vi "Kiwi_Get_Set_Refnum.vi"(8 "error in (no error)":errorcluster, 9 "menu":T11=enum."get", 10 "refnum name":string, 11 "Kiwi DevRef In":T1={"Motor A"={"DeviceStatus"={"status"=FALSE, "code"=0, "source"=""}, "Type"=enum."PWM", "PWM"={"PWM Channel"=enum."Invalid", "DeadBand"={"Name"="", "maxPositivePwm"=0, "minPositivePwm"=0, "centerPwm"=0, "maxNegativePwm"=0, "minNegativePwm"=0, "angularRange"=0}}, "CAN"={"Device Number"=0, "Control Mode"=enum."Percent VBus", "Semaphore"=refnum, "Max Vout"=12.0, "TalonSRX Control Mode"=enum."Percent VBus"}, "Invert"=FALSE}, "Motor B"={"DeviceStatus"={"status"=FALSE, "code"=0, "source"=""}, "Type"=enum."PWM", "PWM"={"PWM Channel"=enum."Invalid", "DeadBand"={"Name"="", "maxPositivePwm"=0, "minPositivePwm"=0, "centerPwm"=0, "maxNegativePwm"=0, "minNegativePwm"=0, "angularRange"=0}}, "CAN"={"Device Number"=0, "Control Mode"=enum."Percent VBus", "Semaphore"=refnum, "Max Vout"=12.0, "TalonSRX Control Mode"=enum."Percent VBus"}, "Invert"=FALSE}, "Motor C"={"DeviceStatus"={"status"=FALSE, "code"=0, "source"=""}, "Type"=enum."PWM", "PWM"={"PWM Channel"=enum."Invalid", "DeadBand"={"Name"="", "maxPositivePwm"=0, "minPositivePwm"=0, "centerPwm"=0, "maxNegativePwm"=0, "minNegativePwm"=0, "angularRange"=0}}, "CAN"={"Device Number"=0, "Control Mode"=enum."Percent VBus", "Semaphore"=refnum, "Max Vout"=12.0, "TalonSRX Control Mode"=enum."Percent VBus"}, "Invert"=FALSE}, "Config Consts"={"Arx"=0.0, "Ay"=0.0, "Brx"=0.0, "By"=0.0, "Cr"=0.0, "Cy"=0.0, "Cx"=0.0, "MaxMotorVal"=0.0}, "status"={"status"=FALSE, "code"=0, "source"=""}, "Angles"={"Angle A"=60.0, "Angle B"=60.0, "Angle C"=60.0, "Radians?"=FALSE}, "MotorVals"={"MotorA"=0.0, "MotorB"=0.0, "MotorC"=0.0}}) -> (0 "error out":errorcluster, 2 "Kiwi DevRef Out":T1={"Motor A"={"DeviceStatus"={"status"=FALSE, "code"=0, "source"=""}, "Type"=enum."PWM", "PWM"={"PWM Channel"=enum."Invalid", "DeadBand"={"Name"="", "maxPositivePwm"=0, "minPositivePwm"=0, "centerPwm"=0, "maxNegativePwm"=0, "minNegativePwm"=0, "angularRange"=0}}, "CAN"={"Device Number"=0, "Control Mode"=enum."Percent VBus", "Semaphore"=refnum, "Max Vout"=12.0, "TalonSRX Control Mode"=enum."Percent VBus"}, "Invert"=FALSE}, "Motor B"={"DeviceStatus"={"status"=FALSE, "code"=0, "source"=""}, "Type"=enum."PWM", "PWM"={"PWM Channel"=enum."Invalid", "DeadBand"={"Name"="", "maxPositivePwm"=0, "minPositivePwm"=0, "centerPwm"=0, "maxNegativePwm"=0, "minNegativePwm"=0, "angularRange"=0}}, "CAN"={"Device Number"=0, "Control Mode"=enum."Percent VBus", "Semaphore"=refnum, "Max Vout"=12.0, "TalonSRX Control Mode"=enum."Percent VBus"}, "Invert"=FALSE}, "Motor C"={"DeviceStatus"={"status"=FALSE, "code"=0, "source"=""}, "Type"=enum."PWM", "PWM"={"PWM Channel"=enum."Invalid", "DeadBand"={"Name"="", "maxPositivePwm"=0, "minPositivePwm"=0, "centerPwm"=0, "maxNegativePwm"=0, "minNegativePwm"=0, "angularRange"=0}}, "CAN"={"Device Number"=0, "Control Mode"=enum."Percent VBus", "Semaphore"=refnum, "Max Vout"=12.0, "TalonSRX Control Mode"=enum."Percent VBus"}, "Invert"=FALSE}, "Config Consts"={"Arx"=0.0, "Ay"=0.0, "Brx"=0.0, "By"=0.0, "Cr"=0.0, "Cy"=0.0, "Cx"=0.0, "MaxMotorVal"=0.0}, "status"={"status"=FALSE, "code"=0, "source"=""}, "Angles"={"Angle A"=60.0, "Angle B"=60.0, "Angle C"=60.0, "Radians?"=FALSE}, "MotorVals"={"MotorA"=0.0, "MotorB"=0.0, "MotorC"=0.0}}, 3 "refnum names":string[](array[string]))   [LabVIEW 2015]
uses:
  <vilib>/Rock Robotics/WPI/Utilities/Refnum Registry Operation.ctl
  <userlib>/836-Library/Drive/kiwi/support/Kiwi_Dev_Ref.ctl
  <vilib>/Rock Robotics/WPI/MotorControl/WPI_MotorControlDeviceRef.ctl
  <vilib>/Rock Robotics/WPI/MotorControl/WPI_MotorControlType.ctl
  <vilib>/Rock Robotics/SystemInterfaces/DIO/FPGA_DIOPWMChannel.ctl
  <vilib>/Rock Robotics/WPI/PWM/WPI_PWMDeadband.ctl
  <vilib>/Rock Robotics/WPI/CAN/Jaguar/SubVIs/WPI_CANJaguar_ControlMode.ctl
  <vilib>/Rock Robotics/WPI/CAN/TalonSRX/WPI_CANTalonSRX_APIControlMode.ctl
  <userlib>/836-Library/Drive/kiwi/support/Kiwi_Cal_Constants.ctl
  <userlib>/836-Library/Drive/kiwi/support/Kiwi_Angles.ctl
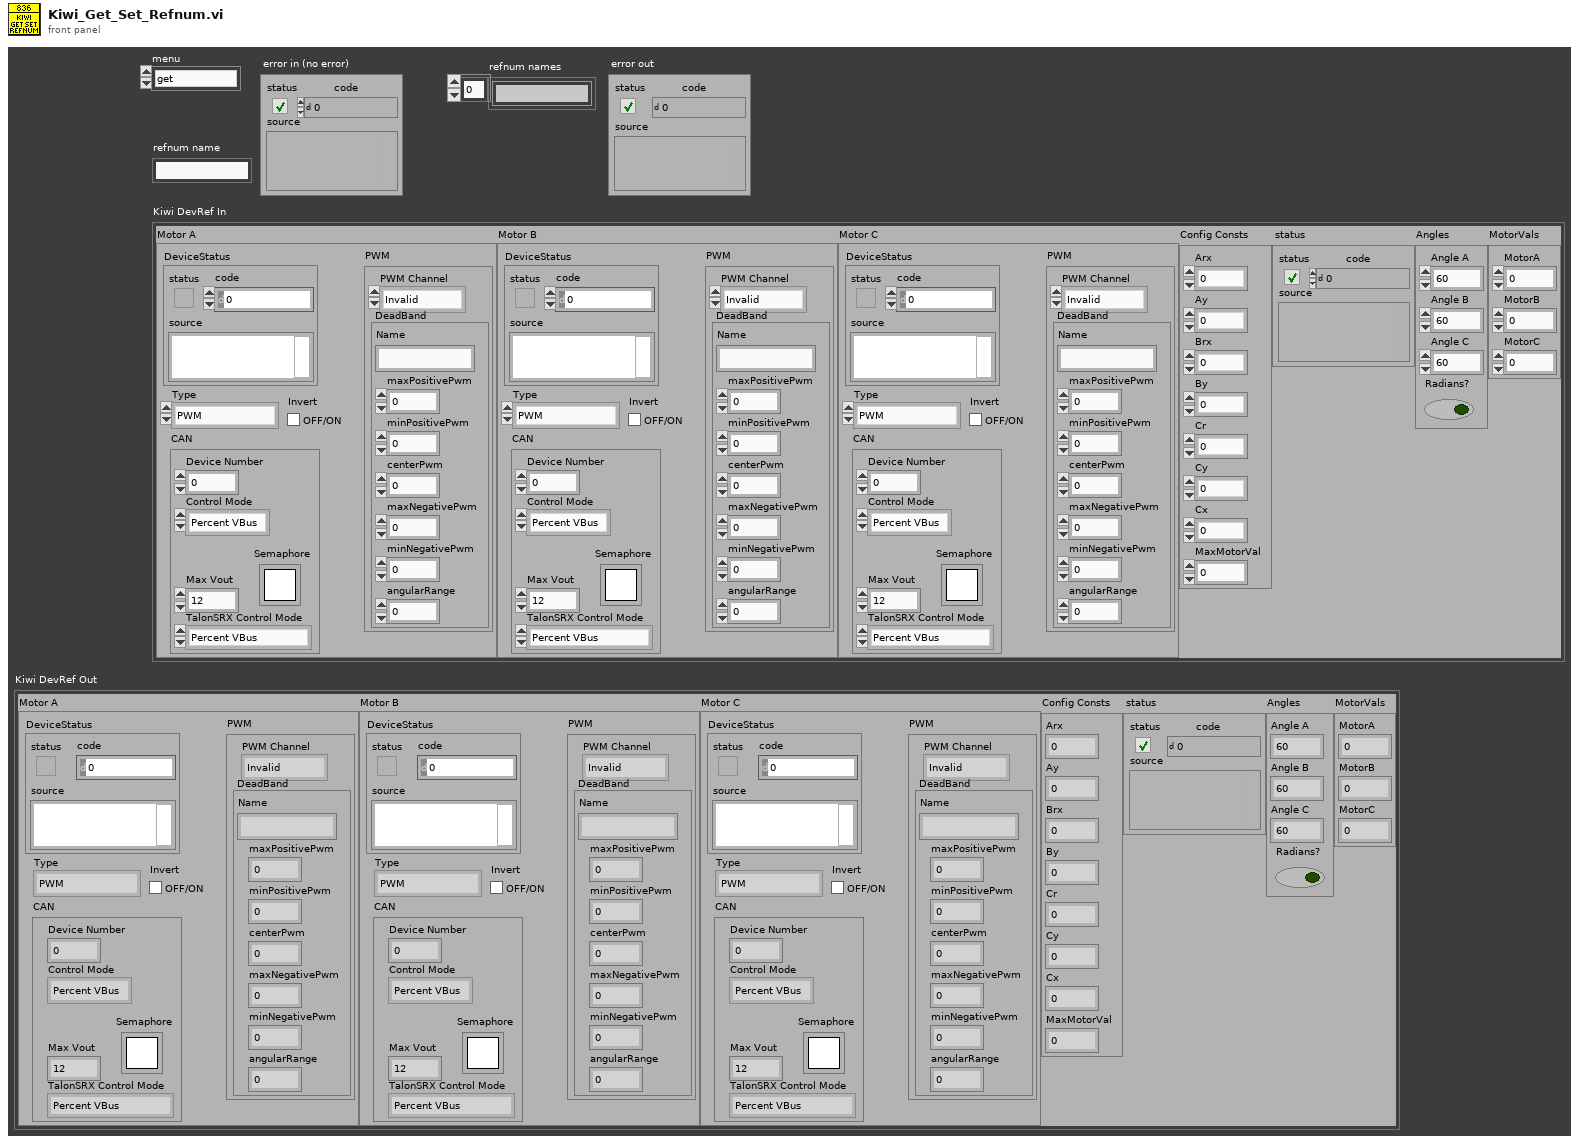
[diagram p1: front panel]
types:
  T1 = typedef "Kiwi_Dev_Ref.ctl" = cluster{"Motor A":T2, "Motor B":T2, "Motor C":T2, "Config Consts":T9, "status":errorcluster, "Angles":T10, "MotorVals":cluster{"MotorA":dbl, "MotorB":dbl, "MotorC":dbl}}
  T2 = typedef "WPI_MotorControlDeviceRef.ctl" = cluster{"DeviceStatus":errorcluster, "Type":T3, "PWM":cluster{"PWM Channel":T4, "DeadBand":T5}, "CAN":cluster{"Device Number":u8, "Control Mode":T6, "Semaphore":T7, "Max Vout":dbl, "TalonSRX Control Mode":T8}, "Invert":bool}
  T3 = typedef "WPI_MotorControlType.ctl" = enum16{"PWM", "CAN", "CANTalonSRX"}
  T4 = typedef "FPGA_DIOPWMChannel.ctl" = enum8{"PWM 0", "PWM 1", "PWM 2", "PWM 3", "PWM 4", "PWM 5", "PWM 6", "PWM 7", "PWM 8", "PWM 9", "PWM MXP 0", "PWM MXP 1", "PWM MXP 2", "PWM MXP 3", "PWM MXP 4", "PWM MXP 5", "PWM MXP 6", "PWM MXP 7", "PWM MXP 8", "PWM MXP 9", "Invalid"}
  T5 = typedef "WPI_PWMDeadband.ctl" = cluster{"Name":string, "maxPositivePwm":i32, "minPositivePwm":i32, "centerPwm":i32, "maxNegativePwm":i32, "minNegativePwm":i32, "angularRange":u16}
  T6 = typedef "WPI_CANJaguar_ControlMode.ctl" = enum8{"Percent VBus", "Current", "Speed", "Position", "Voltage"}
  T7 = typedef "Semaphore RefNum" = refnum<k1>
  T8 = typedef "WPI_CANTalonSRX_APIControlMode.ctl" = enum8{"Percent VBus", "Speed", "Position", "Slave", "Unchanged / Invalid", "Voltage Compensation", "Current", "Motion Profile"}
  T9 = typedef "Kiwi_Cal_Constants.ctl" = cluster{"Arx":dbl, "Ay":dbl, "Brx":dbl, "By":dbl, "Cr":dbl, "Cy":dbl, "Cx":dbl, "MaxMotorVal":dbl}
  T10 = typedef "Kiwi_Angles.ctl" = cluster{"Angle A":dbl, "Angle B":dbl, "Angle C":dbl, "Radians?":bool}
  T11 = typedef "Refnum Registry Operation.ctl" = enum16{"set", "get", "delete", "get all names", "read name"}
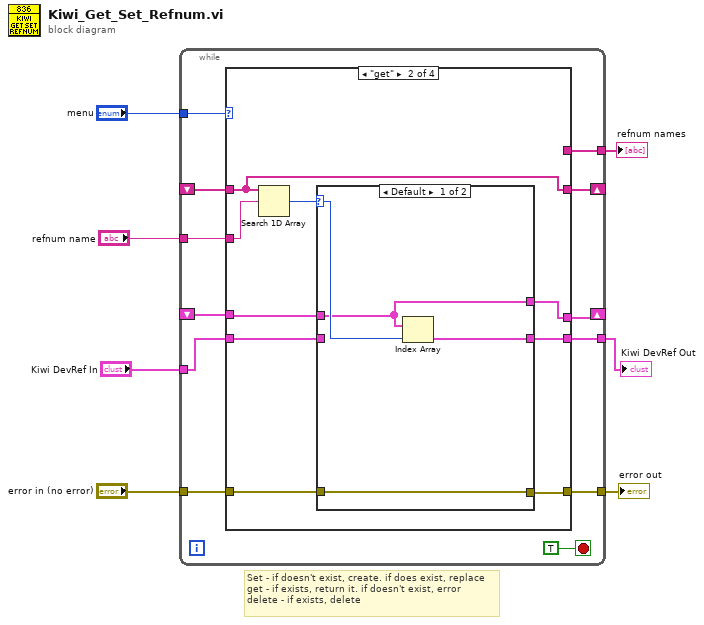
[diagram p0: block diagram]
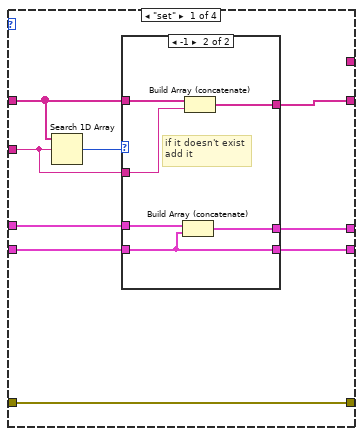
[diagram p2: hidden frame]
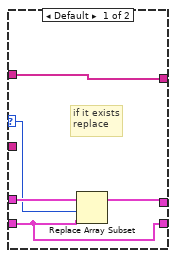
[diagram p3: hidden frame]
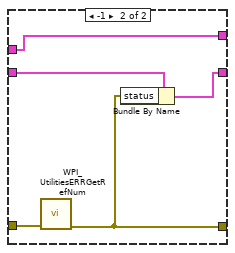
[diagram p4: hidden frame]
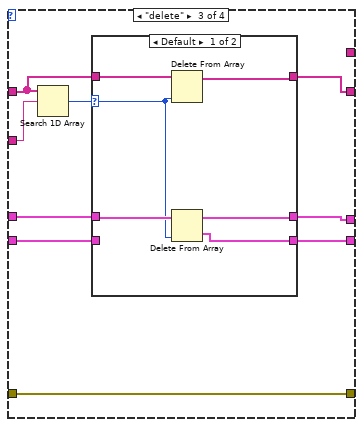
[diagram p5: hidden frame]
diagram:
  # "Set - if doesn't exist, create. if does exist, replace\nget - if exists, return it. if doesn't exist, error\ndelete - if exists, delete"
  n1 = while {
    tunnel: "menu" -> [w18]
    tunnel: "Kiwi DevRef In" -> [w11]
    tunnel: "refnum name" -> [w15]
    tunnel: "error in (no error)" -> [w16]
    shift-right: [w13] -> _
    shift-left: _ -> [w14]
    shift-right: [w9] -> _
    shift-left: _ -> [w12]
    tunnel: [w17] -> w3
    tunnel: [w10] -> w2
    tunnel: [w8] -> w1
    stop <- TRUE stop-if-true
    n2 = case shown="\"get\"" w18 {
      tunnel: [w21 w40 w66 w79] -> w17
      tunnel: w16 -> [w21 w42 w66 w79]
      tunnel: w15 -> [w28 w48 w65 _]
      tunnel: w14 -> [w20 w46 w62 w78]
      tunnel: [w27 w46 w63 w78] -> w13
      tunnel: w12 -> [w25 w45 w60 w77]
      tunnel: w11 -> [w24 w41 w58 w76]
      tunnel: [w23 w44 w59 w76] -> w10
      tunnel: [w22 w43 w61 w77] -> w9
      tunnel: [_ _ _ w78] -> w8
      frame "set" {
        n3 = Search 1D Array(1D array=w20, element=w28) -> (index of element=w26:i32)  [unwired: 1 in]
        n4 = case shown="-1" w26 {
          selector: w26 -> [w31 _]
          tunnel: w20 -> [w33 w39]
          tunnel: w28 -> [_ w38]
          tunnel: [w33 w37] -> w27
          tunnel: w25 -> [w32 w36]
          tunnel: w24 -> [w29 w35]
          tunnel: [w29 w35] -> w23
          tunnel: [w30 w34] -> w22
          frame Default {
            # "if it exists\nreplace"
            n5 = Replace Array Subset(array=w32, new element=w29, index=w31) -> (w30:T1[])
          }
          frame -1 {
            # "if it doesn't exist\nadd it"
            n6 = Build Array (concatenate)(w36, w35) -> (w34:T1[])
            n7 = Build Array (concatenate)(w39, w38) -> (w37:string[])
          }
        }
      }
      frame "get" {
        n8 = Search 1D Array(1D array=w46, element=w48) -> (index of element=w47:i32)  [unwired: 1 in]
        n9 = case shown="Default" w47 {
          selector: w47 -> [w52 _]
          tunnel: w45 -> [w50 w53]
          tunnel: [w51 w54] -> w44
          tunnel: [w50 w53] -> w43
          tunnel: w42 -> [w49 w57]
          tunnel: w41 -> [_ w56]
          tunnel: [w49 w55] -> w40
          frame Default {
            n10 = Index Array(array=w50, index=w52) -> (element=w51:T1)
          }
          frame -1 {
            n11 = call <vilib>:"WPI_UtilitiesERRGetRefNum.vi"("error in (no error)"=w57) -> ("ERRGetRefNum"=w55:errorcluster)  [unwired: 10 out]
            n12 = Bundle By Name(cluster=w56, "status"=w55) -> (w54:T1)
          }
        }
      }
      frame "delete" {
        n13 = Search 1D Array(1D array=w62, element=w65) -> (index of element=w64:i32)  [unwired: 1 in]
        n14 = case shown="Default" w64 {
          selector: w64 -> [w70 _]
          tunnel: [w67 w75] -> w63
          tunnel: w62 -> [w72 w75]
          tunnel: [w69 w74] -> w61
          tunnel: w60 -> [w71 w74]
          tunnel: [w68 w73] -> w59
          tunnel: w58 -> [_ w73]
          frame Default {
            n15 = Delete From Array(array=w72, index=w70) -> (array with subset deleted=w67:string[])  [unwired: 1 in, 1 out]
            n16 = Delete From Array(array=w71, index=w70) -> (deleted portion=w68:T1, array with subset deleted=w69:T1[])  [unwired: 1 in]
          }
          frame -1 {
          }
        }
      }
      frame "get all names", Default {
      }
    }
  }
  "Kiwi DevRef Out" <- w2
  "error out" <- w3
  "refnum names" <- w1
